vi "Rotational and Translational Drive.vi"(8 "error in":errorcluster, 9 "Z":dbl, 10 "Y":dbl, 11 "X":dbl) -> (0 "error out":errorcluster)   [LabVIEW 2016]
uses:
  Refname/Motors.ctl
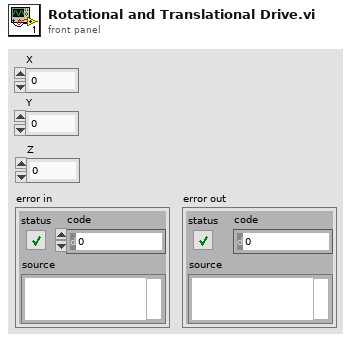
[diagram p1: front panel]
types:
  T1 = typedef "Motors.ctl" = enum16{"Wheel 1", "Swerve 1", "Wheel 2", "Swerve 2", "Wheel 3", "Swerve 3", "Wheel 4", "Swerve 4"}
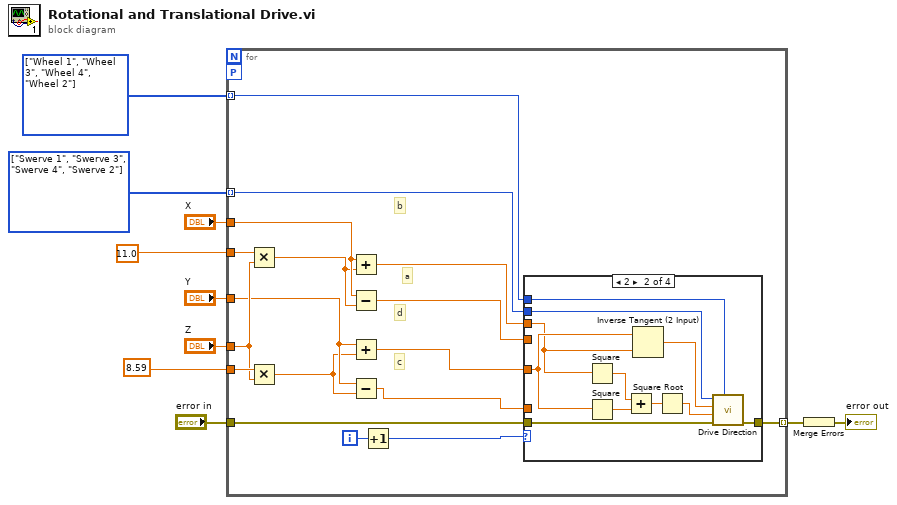
[diagram p0: block diagram]
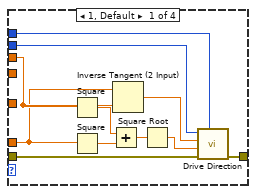
[diagram p2: hidden frame]
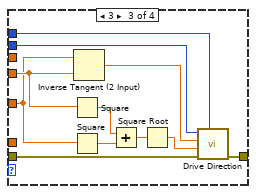
[diagram p3: hidden frame]
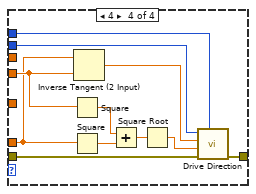
[diagram p4: hidden frame]
diagram:
  w10 = T1[] [enum."Swerve 1", enum."Swerve 3", enum."Swerve 4", enum."Swerve 2"] items=["Wheel 1", "Swerve 1", "Wheel 2", "Swerve 2", "Wheel 3", "Swerve 3", "Wheel 4", "Swerve 4"]
  w9 = T1[] [enum."Wheel 1", enum."Wheel 3", enum."Wheel 4", enum."Wheel 2"] items=["Wheel 1", "Swerve 1", "Wheel 2", "Swerve 2", "Wheel 3", "Swerve 3", "Wheel 4", "Swerve 4"]
  n1 = for {
    workers-P: _ -> [_]
    tunnel: w10 -> [w14] mode=indexing
    tunnel: w9 -> [w13] mode=indexing
    tunnel: 11.0 -> [w25]
    tunnel: 8.59 -> [w27]
    tunnel: "X" -> [w24]
    tunnel: "Y" -> [w22]
    tunnel: "Z" -> [w26]
    tunnel: "error in" -> [w12]
    tunnel: [w11] -> w2 mode=indexing
    i -> [w20]
    # "d"
    # "c"
    # "b"
    # "a"
    n2 = Multiply(x=w25, y=w26) -> (x*y=w23:dbl)
    n3 = Multiply(x=w27, y=w26) -> (x*y=w21:dbl)
    n4 = Add(x=w24, y=w23) -> (x+y=w17:dbl)
    n5 = Subtract(x=w24, y=w23) -> (x-y=w18:dbl)
    n6 = Add(x=w22, y=w21) -> (x+y=w15:dbl)
    n7 = Subtract(x=w22, y=w21) -> (x-y=w16:dbl)
    n8 = Increment(x=w20) -> (x+1=w19:i32)
    n9 = case shown="2" w19 {
      tunnel: w18 -> [_ _ w55 w66]
      tunnel: w17 -> [w34 w43 _ _]
      tunnel: w16 -> [w29 _ _ w65]
      tunnel: w15 -> [_ w44 w54 _]
      tunnel: w14 -> [w32 w40 w51 w62]
      tunnel: w13 -> [w31 w41 w52 w63]
      tunnel: w12 -> [w30 w42 w53 w64]
      tunnel: [w28 w39 w50 w61] -> w11
      frame 1, Default {
        n10 = Square(x=w34) -> (x^2=w38:dbl)
        n11 = Square(x=w29) -> (x^2=w37:dbl)
        n12 = Add(x=w38, y=w37) -> (x+y=w36:dbl)
        n13 = Inverse Tangent (2 Input)(1:w34, 2:w29) -> (0:w33:dbl)
        n14 = Square Root(x=w36) -> (sqrt(x)=w35:dbl)
        n15 = call "Drive Direction.vi"("Wheels"=w31, "error in"=w30, "Wheel Power"=w35, "Desired direction (radians)"=w33, "Swerve"=w32) -> ("error out"=w28:errorcluster)  [unwired: 6 in]
      }
      frame 2 {
        n16 = Square(x=w43) -> (x^2=w49:dbl)
        n17 = Square(x=w44) -> (x^2=w48:dbl)
        n18 = Add(x=w49, y=w48) -> (x+y=w47:dbl)
        n19 = Inverse Tangent (2 Input)(1:w43, 2:w44) -> (0:w45:dbl)
        n20 = Square Root(x=w47) -> (sqrt(x)=w46:dbl)
        n21 = call "Drive Direction.vi"("Wheels"=w41, "error in"=w42, "Wheel Power"=w46, "Desired direction (radians)"=w45, "Swerve"=w40) -> ("error out"=w39:errorcluster)  [unwired: 6 in]
      }
      frame 3 {
        n22 = Square(x=w55) -> (x^2=w56:dbl)
        n23 = Square(x=w54) -> (x^2=w57:dbl)
        n24 = Inverse Tangent (2 Input)(1:w55, 2:w54) -> (0:w60:dbl)
        n25 = Add(x=w56, y=w57) -> (x+y=w58:dbl)
        n26 = Square Root(x=w58) -> (sqrt(x)=w59:dbl)
        n27 = call "Drive Direction.vi"("Wheels"=w52, "error in"=w53, "Wheel Power"=w59, "Desired direction (radians)"=w60, "Swerve"=w51) -> ("error out"=w50:errorcluster)  [unwired: 6 in]
      }
      frame 4 {
        n28 = Square(x=w66) -> (x^2=w67:dbl)
        n29 = Square(x=w65) -> (x^2=w68:dbl)
        n30 = Inverse Tangent (2 Input)(1:w66, 2:w65) -> (0:w71:dbl)
        n31 = Add(x=w67, y=w68) -> (x+y=w69:dbl)
        n32 = Square Root(x=w69) -> (sqrt(x)=w70:dbl)
        n33 = call "Drive Direction.vi"("Wheels"=w63, "error in"=w64, "Wheel Power"=w70, "Desired direction (radians)"=w71, "Swerve"=w62) -> ("error out"=w61:errorcluster)  [unwired: 6 in]
      }
    }
  }
  n34 = Merge Errors(w2) -> (→"error out":errorcluster)
